vi "Suite.vi"(8 "error in (no error)":errorcluster, 11 "LUnit Test Case in":refnum<class "LUnit Inheriting Test Case.lvclass">) -> (0 "error out":errorcluster, 2 "LUnit Test Suite Out":refnum<class "LUnit Test Suite.lvclass">, 3 "LUnit Test Case out":refnum<class "LUnit Inheriting Test Case.lvclass">)   [LabVIEW 2020, in "LUnit Inheriting Test Case.lvclass"]
uses:
  LUnit Inheriting Test Case.lvclass
  C:/git/astemes-lunit/source/API/LUnit Test Case/LUnit Test Case.lvclass
  C:/git/astemes-lunit/source/Core/Runnable/Runnable.lvclass
  LUnit Test Suite/LUnit Test Suite.lvclass
  LUnit Test Case/LUnit Test Case.lvclass/LUnit Test Case.ctl
  <vilib>/Utility/LVClass/Get LV Class Name.vi
  LUnit Test Case/LUnit Test Case.lvclass
  LUnit Inheriting Test Case.lvclass/LUnit Inheriting Test Case.ctl
  C:/git/astemes-lunit/source/API/LUnit Inheriting Test Case/LUnit Test Case/LUnit Inheriting Test Case.lvclass
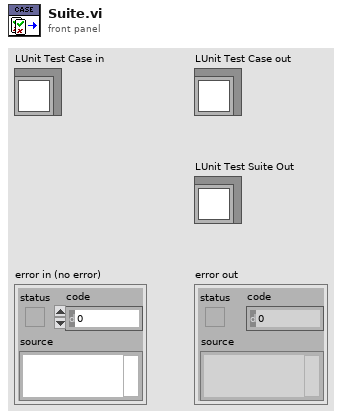
[diagram p1: front panel]
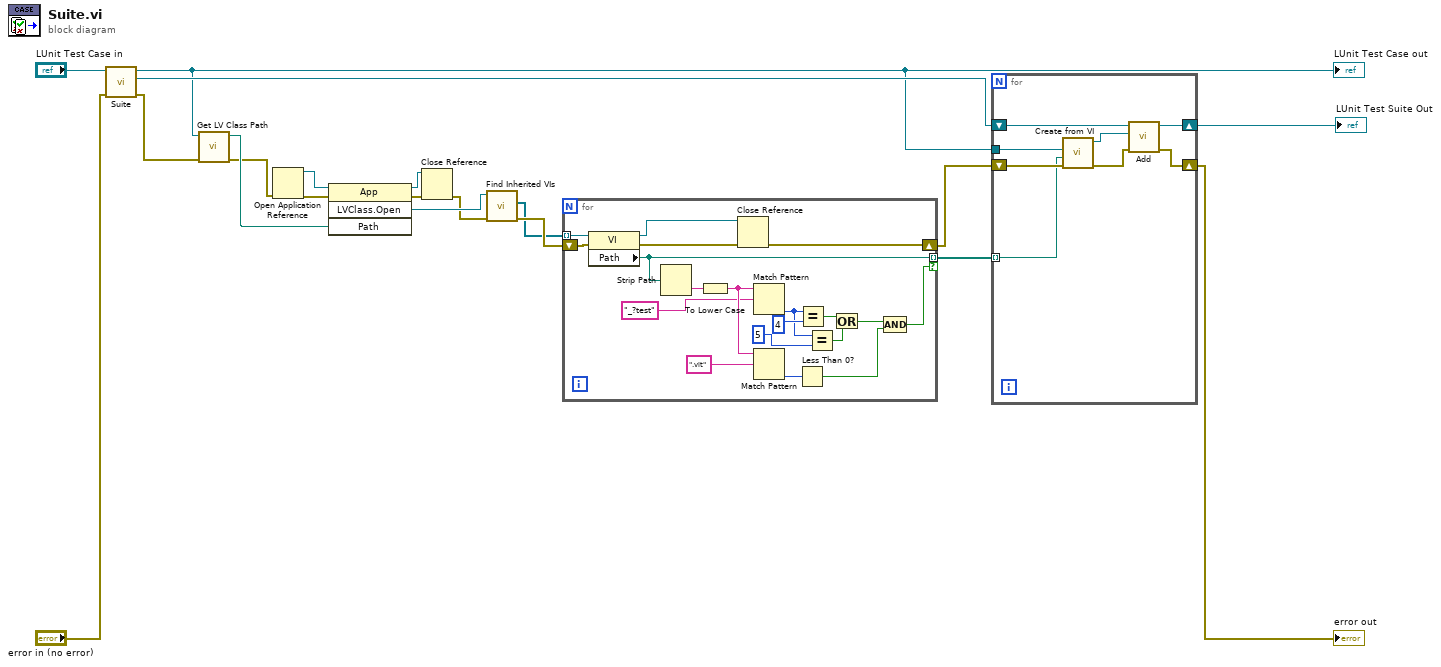
[diagram p0: block diagram]
diagram:
  n1 = call-parent "Suite.vi"("error in (no error)"="error in (no error)", "LUnit Test Case in"="LUnit Test Case in") -> ("error out"=w4:errorcluster, "LUnit Test Suite Out"=w3:refnum<class "LUnit Test Suite.lvclass">, "LUnit Test Case out"=w1:refnum<class "LUnit Inheriting Test Case.lvclass">)  [unwired: 7 in]
  "LUnit Test Case out" <- w1
  n2 = call <vilib>:"Get LV Class Path.vi"("error in (no error)"=w4, "object"=w1) -> ("error out"=w8:errorcluster, "class path"=w9:path)  [unwired: 8 in]
  n3 = Open Application Reference(8:w8) -> (0:w17:errorcluster, 3:w18:refnum<vi>)  [unwired: 3 in]
  n4 = invoke class="App" method="LVClass.Open"(reference=w18, error in=w17, "Path"=w9) -> (reference out=w14:refnum<vi>, error out=w16:errorcluster, "LVClass.Open"=w13:refnum<vi>)  [unwired: 1 in, 1 out]
  n5 = Close Reference(reference=w14, error in (no error)=w16) -> (error out=w10:errorcluster)
  n6 = call "Find Inherited VIs.vi"("error in (no error)"=w10, "LVClassLibrary in"=w13) -> ("error out"=w12:errorcluster, "Inherited Dynamic Member VIs"=w2:refnum<vi>[])  [unwired: 8 in]
  n7 = for {
    tunnel: w2 -> [w38] mode=indexing
    tunnel: [w33] -> w15 mode=indexing if=w28
    shift-right: [w35] -> w11
    shift-left: w12 -> [w37]
    n8 = property class="VI"(reference=w38, error in=w37) -> (reference out=w34:refnum<vi>, error out=w36:errorcluster, "Path"=w33:path)
    n9 = Strip Path(path=w33) -> (name=w32:string)  [unwired: 1 out]
    n10 = To Lower Case(string=w32) -> (all lower case string=w31:string)
    n11 = Close Reference(reference=w34, error in (no error)=w36) -> (error out=w35:errorcluster)
    n12 = Match Pattern(string=w31, regular expression="_?test") -> (offset past match=w25:i32)  [unwired: 1 in, 3 out]
    n13 = Match Pattern(string=w31, regular expression=".vit") -> (offset past match=w29:i32)  [unwired: 1 in, 3 out]
    n14 = Less Than 0?(x=w29) -> (x < 0?=w27:bool)
    n15 = Equal?(x=w25, y=4) -> (x = y?=w23:bool)
    n16 = Equal?(x=w25, y=5) -> (x = y?=w20:bool)
    n17 = Or(x=w23, y=w20) -> (x .or. y?=w21:bool)
    n18 = Compound Arithmetic op=AND(w21, w27) -> (w28:bool)
  }
  n19 = for {
    tunnel: w15 -> [w41] mode=indexing
    shift-right: [w45] -> w7
    shift-left: w3 -> [w46]
    shift-right: [w43] -> w6
    shift-left: w11 -> [w42]
    tunnel: w1 -> [w39]
    n20 = call "Create from VI.vi"("error in (no error)"=w42, "Test Method VI Path"=w41, "LUnit Test Case Class"=w39) -> ("error out"=w44:errorcluster, "LUnit Test Case"=w40:refnum<class "LUnit Inheriting Test Case.lvclass">)  [unwired: 7 in]
    n21 = call "Add.vi"("error in (no error)"=w44, "Runnable"=w40, "LUnit Test Suite In"=w46) -> ("error out"=w43:errorcluster, "LUnit Test Suite In"=w45:refnum<class "LUnit Test Suite.lvclass">)  [unwired: 7 in]
  }
  "error out" <- w6
  "LUnit Test Suite Out" <- w7
